vi "插值拟合切线.vi"(4 "计算参数 in":T2, 5 "输入参数 in":T1, 7 "Array in":dbl[](array[numeric])) -> (0 "计算参数 out":T2, 1 "输入参数 out":T1, 3 "Array out":dbl[](array[numeric]))   [LabVIEW 2013]
doc: "插值拟合得到切线，取95%-60%之间每5%取一个点，计算最小二乘拟合直线，获得直线的斜率和截距"
uses:
  <vilib>/Analysis/NI_AALPro.lvlib
panel:
  out "数组 2":dbl[](array[numeric])
  out "y%":dbl[](array[numeric])
  out "X":dbl[](array[numeric])
  out "Y":dbl[](array[numeric])
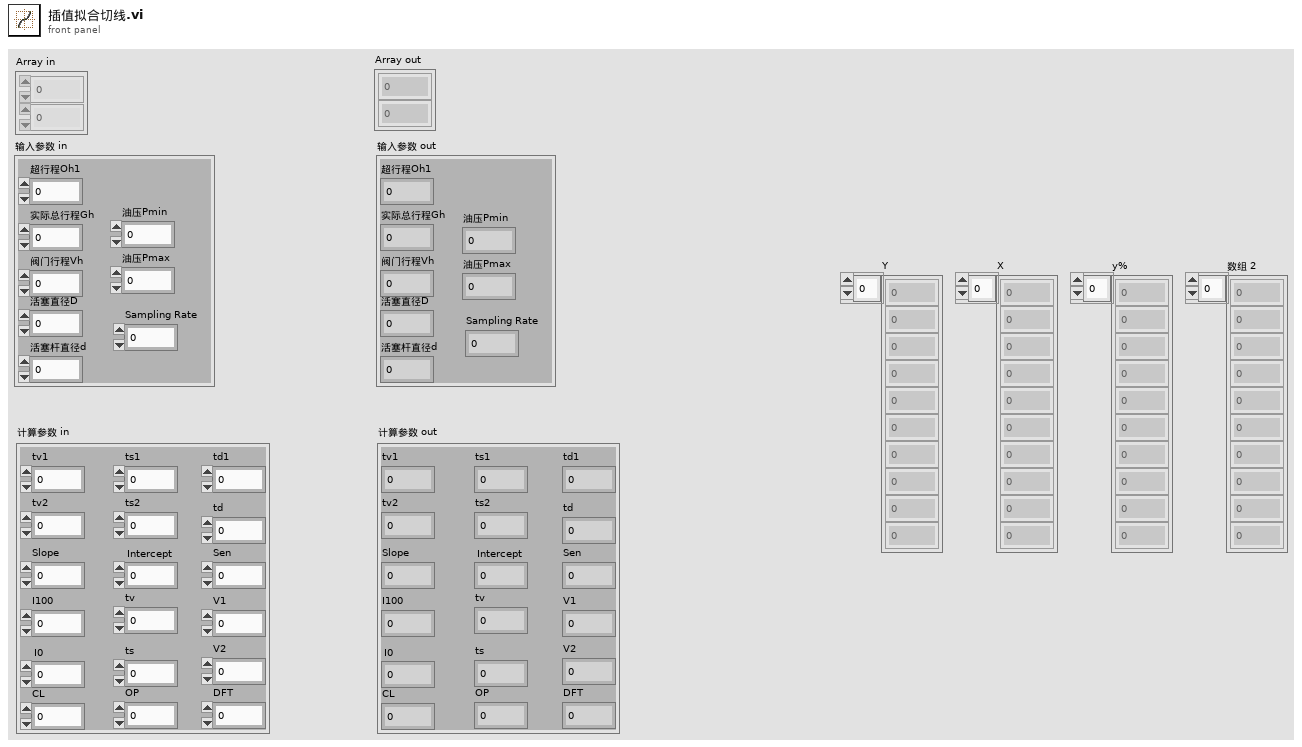
[diagram p1: front panel]
types:
  T1 = cluster{"超行程Oh1":dbl, "实际总行程Gh":dbl, "阀门行程Vh":dbl, "活塞直径D":dbl, "活塞杆直径d":dbl, "油压Pmin":dbl, "油压Pmax":dbl, "Sampling Rate":dbl}
  T2 = cluster{"tv1":dbl, "tv2":dbl, "tv":dbl, "ts1":dbl, "ts2":dbl, "ts":dbl, "td1":dbl, "td":dbl, "Slope":dbl, "Intercept":dbl, "I100":dbl, "I0":dbl, "Sen":dbl, "V1":dbl, "V2":dbl, "CL":dbl, "OP":dbl, "DFT":dbl}
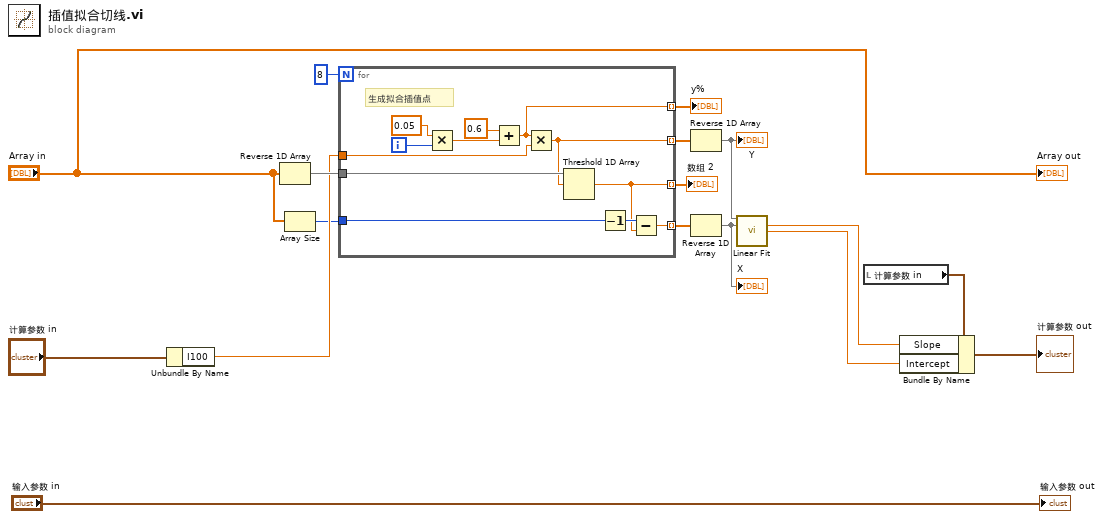
[diagram p0: block diagram]
diagram:
  n1 = Unbundle By Name("计算参数 in") -> ("I100"=w4:dbl)
  n2 = Reverse 1D Array(array="Array in") -> (reversed array=w13:dbl[])
  n3 = Array Size(array="Array in") -> (size(s)=w3:i32)
  n4 = for {
    N: 8 -> [_]
    tunnel: [w24] -> w16 mode=indexing
    tunnel: w13 -> [w25]
    tunnel: [w22] -> w14 mode=indexing
    tunnel: w4 -> [w23]
    tunnel: w3 -> [w20]
    tunnel: [w21] -> w11 mode=indexing
    tunnel: [w18] -> w10 mode=indexing
    i -> [w27]
    # "生成拟合插值点"
    n5 = Multiply(x=0.05, y=w27) -> (x*y=w28:dbl)
    n6 = Add(x=0.6, y=w28) -> (x+y=w21:dbl)
    n7 = Multiply(x=w21, y=w23) -> (x*y=w24:dbl)
    n8 = Threshold 1D Array(2:w24, 3:w25) -> (0:w18:dbl)  [unwired: 1 in]
    n9 = Decrement(x=w20) -> (x-1=w19:i32)
    n10 = Subtract(x=w19, y=w18) -> (x-y=w22:dbl)
  }
  "y%" <- w11
  "数组 2" <- w10
  n11 = Reverse 1D Array(array=w16) -> (reversed array=w17:dbl[])
  "Y" <- w17
  n12 = Reverse 1D Array(array=w14) -> (reversed array=w15:dbl[])
  "X" <- w15
  n13 = call <vilib>:"Linear Fit.vi"("Y"=w17, "X"=w15) -> ("slope"=w5:dbl, "intercept"=w6:dbl)  [unwired: 9 in, 3 out]
  n14 = local read "计算参数 in"() -> (w7:T2)
  n15 = Bundle By Name(cluster=w7, "Slope"=w5, "Intercept"=w6) -> (→"计算参数 out":T2)
  "Array out" <- "Array in"
  "输入参数 out" <- "输入参数 in"
